vi "M2因子计算.vi"(8 "method":T1 items=["Least Square", "Least Absolute Residual", "Bisquare"], 9 "位置":dbl[](array[numeric]), 10 "光斑半径":dbl[](array[numeric]), 11 "激光波长":dbl) -> (3 "M2因子":dbl)   [LabVIEW 2015]
uses:
  <vilib>/Analysis/6fits.llb/Curve Fitting Criteria.ctl
  <vilib>/Analysis/NI_AALPro.lvlib
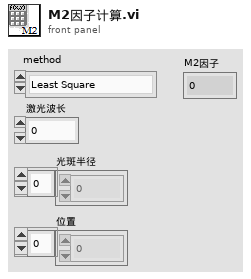
[diagram p1: front panel]
types:
  T1 = typedef "NI_AALPro.lvlib/Curve Fitting Criteria.ctl" = u16
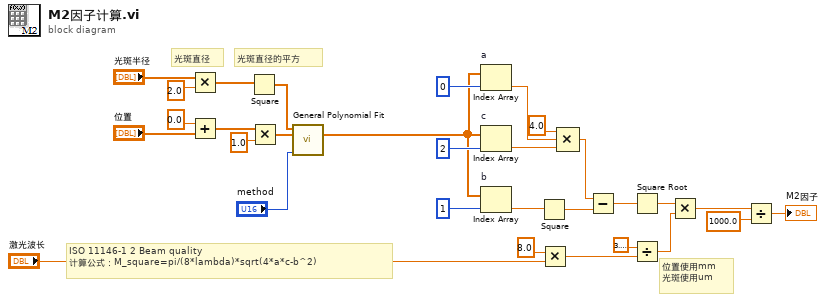
[diagram p0: block diagram]
diagram:
  # "位置使用mm\n光斑使用um"
  # "ISO 11146-1 2 Beam quality\n计算公式：M_square=pi/(8*lambda)*sqrt(4*a*c-b^2)"
  # "光斑直径的平方"
  # "光斑直径"
  n1 = Multiply(x="光斑半径", y=2.0) -> (x*y=w26:dbl[])
  n2 = Add(x=0.0, y="位置") -> (x+y=w29:dbl[])
  n3 = Square(x=w26) -> (x^2=w25:dbl[])
  n4 = Multiply(x=w29, y=1.0 ("x")) -> (x*y=w24:dbl[])
  n5 = call <vilib>:"General Polynomial Fit.vi"("Y"=w25, "X"=w24, "method"="method") -> ("Polynomial Coefficients"=w6:dbl[])  [unwired: 9 in, 3 out]
  n6 = Index Array "a"(array=w6, index=0) -> (element=w19:dbl)
  n7 = Index Array "c"(array=w6, index=2) -> (element=w7:dbl)
  n8 = Index Array "b"(array=w6, index=1) -> (element=w18:dbl)
  n9 = Square(x=w18) -> (x^2=w16:dbl)
  n10 = Multiply(x=8.0, y="激光波长") -> (x*y=w13:dbl)
  n11 = Compound Arithmetic op=MULTIPLY(4.0 ("value"), w19, w7) -> (w17:dbl)
  n12 = Subtract(x=w17, y=w16) -> (x-y=w15:dbl)
  n13 = Square Root(x=w15) -> (sqrt(x)=w10:dbl)
  n14 = Divide(x=3.141592653589793, y=w13) -> (x/y=w11:dbl)
  n15 = Multiply(x=w10, y=w11) -> (x*y=w9:dbl)
  n16 = Divide(x=w9, y=1000.0) -> (x/y=→"M2因子":dbl)
